vi "Driver Get.vi"(8 "error in (no error)":errorcluster, 9 "sType":string, 10 "sxDriverId":string, 11 "Connection Refnum":T1) -> (0 "error out":errorcluster, 2 "Driver Record":T2, 3 "Connection Refnum":T1, 4 "Data Present":bool)   [LabVIEW 2011]
uses:
  Driver Record.ctl
  Summitek EXT/ODBC/SQL Controls/Connection Refnum.ctl
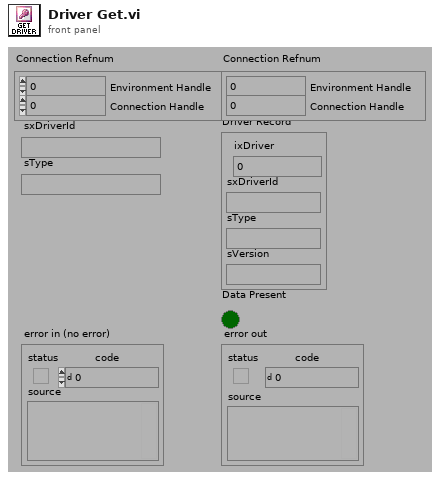
[diagram p1: front panel]
types:
  T1 = typedef "Connection Refnum.ctl" = cluster{"Environment Handle":i32, "Connection Handle":i32}
  T2 = typedef "Driver Record.ctl" = cluster{"ixDriver":i32, "sxDriverId":string, "sType":string, "sVersion":string}
  T3 = typedef "Statement Refnum.ctl" = cluster{"Statement Handle":i32, "Parameter Number":u16}
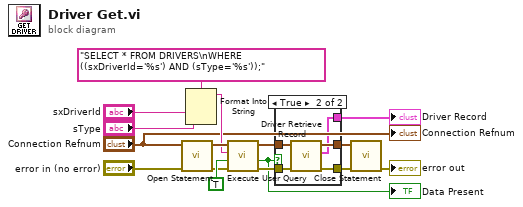
[diagram p0: block diagram]
diagram:
  n1 = call "Open Statement.vi"("error in (no error)"="error in (no error)", "Connection Refnum"="Connection Refnum") -> ("error out"=w8:errorcluster, "Statement Refnum"=w9:T3)  [unwired: 4 out]
  n2 = Format Into String(format string="SELECT * FROM DRIVERS\nWHERE ((sxDriverId='%s') AND (sType='%s'));" ("User Query"), "sxDriverId", "sType") -> (resulting string=w7:string)  [unwired: 2 in, 1 out]
  n3 = call "Execute User Query.vi"("error in (no error)"=w8, "Return Data? (f)"=TRUE, "User Query"=w7, "Statement Refnum"=w9) -> ("error out"=w16:errorcluster, "Data Present?"=w6:bool, "Statement Refnum"=w15:T3)  [unwired: 1 out]
  "Data Present" <- w6
  n4 = case shown="True" w6 {
    tunnel: w16 -> [w17 w22]
    tunnel: w15 -> [w18 w23]
    tunnel: [w17 w20] -> w12
    tunnel: [w18 w21] -> w13
    tunnel: [_ w19] -> w4
    frame False {
    }
    frame True {
      n5 = call "Driver Retrieve Record.vi"("error in (no error)"=w22, "Statement Refnum"=w23) -> ("error out"=w20:errorcluster, "Driver Record"=w19:T2, "Statement Refnum"=w21:T3)  [unwired: 7 out]
    }
  }
  "Driver Record" <- w4
  n6 = call "Close Statement.vi"("error in (no error)"=w12, "Statement Refnum"=w13) -> ("error out"=→"error out":errorcluster)  [unwired: 5 out]
  "Connection Refnum" <- "Connection Refnum"
